vi "HEWH Search Element.vi"(10 "Search Element":string, 11 "Full Data":string[][](array[string])) -> (3 "Data":string)   [LabVIEW 2023]
panel:
  out "index of element":i32
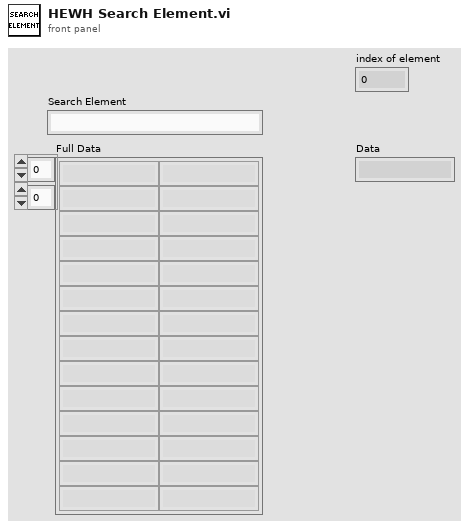
[diagram p1: front panel]
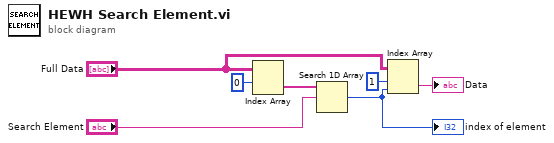
[diagram p0: block diagram]
diagram:
  n1 = Index Array(array="Full Data", index (row)=0 ("index")) -> (element=w2:string[])  [unwired: 1 in]
  n2 = Search 1D Array(1D array=w2, element="Search Element") -> (index of element=w5:i32)  [unwired: 1 in]
  "index of element" <- w5
  n3 = Index Array(array="Full Data", index (row)=1 ("disabled index (row)"), index (col)=w5) -> (element=→"Data":string)
